vi "Counter to DAC.vi"() -> ()   [LabVIEW 2014]
uses:
  <vilib>/Platform/TimedLoop/XDataNode/timing_clust.ctl
  <vilib>/Platform/TimedLoop/XDataNode/nitl_modes.ctl
  <vilib>/Platform/TimedLoop/XDataNode/wakeup.ctl
  <vilib>/rvi/Emulation/niFpgaGetClockAttributes.vi
  <vilib>/rvi/Emulation/niFpgaSctlEmulationGetInTimedLoop.vi
  <vilib>/rvi/Emulation/niFpgaEmulationReportErrorSimple.vi
  <vilib>/rvi/Emulation/niFpgaProcessEmulError.vi
  <vilib>/rvi/Emulation/niFpgaCriticalErrorInLSC.vi
  <vilib>/rvi/interface/RandomDataEmulation/niFpgaRandomDataHandleErrors.vi
  <vilib>/rvi/eio/common/nirviEmuTemplateMethod_errors.vi
  <vilib>/Platform/TimedLoop/XDataNode/XDataNode.xnode
  <vilib>/rvi/DataTransferAndStorage/Container/XNode/niFpgaContainer.xnode
  <vilib>/rvi/interface/RandomDataEmulation/nirviRandomDataFpgaReadWriteTemplate.vi
  <vilib>/eio/EIONode/EIONode.xnode
  <vilib>/Platform/TimedLoop/XDataNode/XDNodeRunTimeDep.lvlib
panel:
  in  "ExtTrigEnable":bool
  in  "FIFOflag":bool
  out "Triggered":bool
  in  "Scale 2":i16=100
  in  "Scale 1":i16=100
  in  "Offset 2":i16
  in  "Offset 1":i16
  in  "Counter ticks":u32=40000
  out "Ctr Elapsed":u32
  out "BlocksTransfered":u32
  out "Ctr Overflow?":bool
  in  "Ctr FIFO":bool
  in  "Outputs\nDIO 12-14":bool[](array[boolean])=[FALSE, FALSE, FALSE, FALSE]
  out "Inputs\nDIO 8-10":bool[](array[boolean])=[TRUE, FALSE, FALSE]
  out "Counts":u32[](array[numeric])
  out "loop elapsed":u16
  in  "Rate":u32=400 caption="Count(Ticks)"
  out "DAC 2":i16
  out "DAC 1":i16
  in  "Dac2 sub":bool[](array[boolean])=[FALSE, FALSE, FALSE, FALSE, FALSE, FALSE, FALSE, FALSE]
  in  "Dac2 add":bool[](array[boolean])=[TRUE, TRUE, TRUE, TRUE, TRUE, TRUE, TRUE, FALSE]
  in  "Dac1 sub":bool[](array[boolean])=[FALSE, FALSE, FALSE, FALSE, FALSE, FALSE, FALSE, FALSE]
  in  "Dac1 add":bool[](array[boolean])=[TRUE, TRUE, TRUE, TRUE, TRUE, TRUE, TRUE, FALSE]
  # "Counter FIFO"
  # "Hz to Volts"
  # "TTL I/O"
  # "FPGA DMA-FIFO CANNOT be cleared by FPGA,\nonly by PC Host VI. Ctr Overflow will be on when\nFPGA-side FIFO is full!"
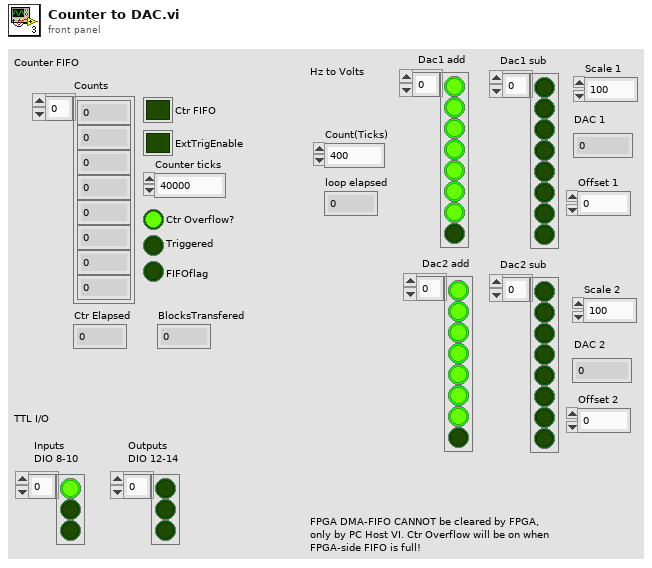
[diagram p1: front panel]
types:
  T1 = typedef "XDNodeRunTimeDep.lvlib/timing_clust.ctl" = cluster{"Expected End [f-1]":u64, "Actual End [f-1]":u64, "Finished Late? [f-1]":bool, "Expected End [i-1]":u64, "Actual End [i-1]":u64, "Finished Late? [i-1]":bool, "Expected Start [i]":u64, "Actual Start [i]":u64, "Expected Start [f]":u64, "Actual Start [f]":u64, "Source Name":string, "Structure Name":string, "Period":i64, "Deadline":i64, "Offset":i64, "Start":i64, "Priority":i32, "Timeout":i32, "Mode":T2, "Wakeup Reason":T3, "Error":errorcluster, "Source Type":string, "Secondary Source Type":string, "Global End Time":u64, "Global Start Time":u64, "Frame Duration":u64, "Iteration Duration":u64, "Assigned CPU":i32, "I/O Scan Engine Mode":u32}
  T2 = typedef "XDNodeRunTimeDep.lvlib/nitl_modes.ctl" = enum32{"No Change", "Process missed periods, maintain original phase", "Discard missed periods, maintain original phase", "Process missed periods, ignore original phase", "Discard missed periods, ignore original phase"}
  T3 = typedef "XDNodeRunTimeDep.lvlib/wakeup.ctl" = enum32{"Normal", "Aborted", "Asynchronous wakeup", "Timing source error", "Timed loop error", "Timeout"}
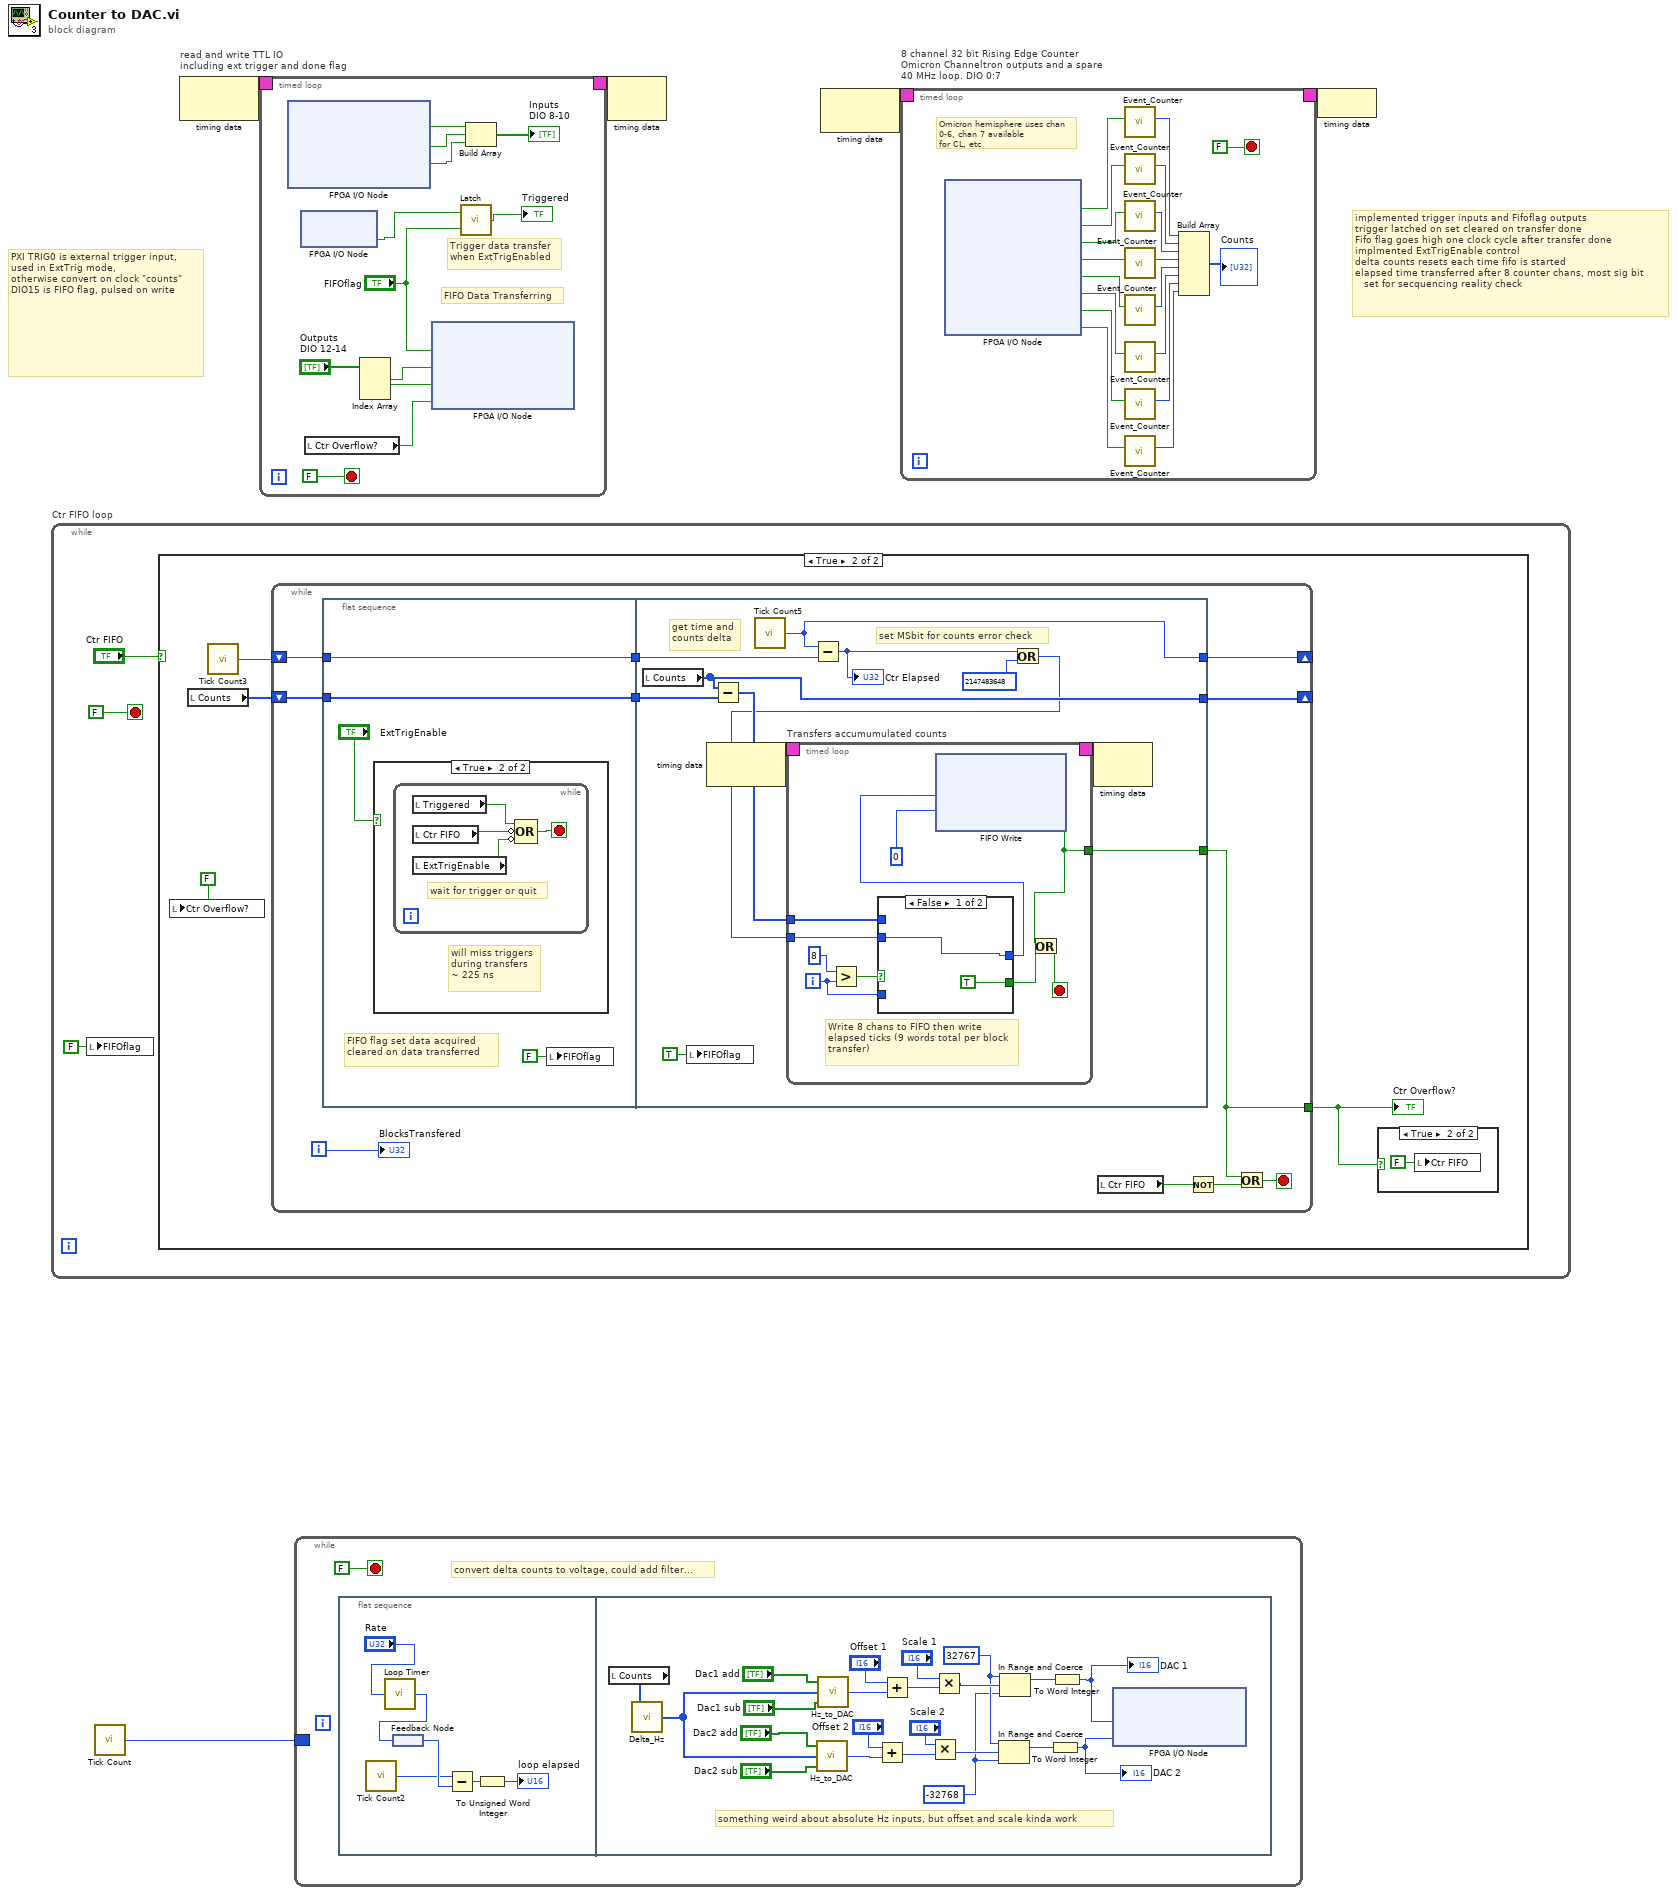
[diagram p0: block diagram]
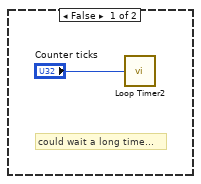
[diagram p4: hidden frame]
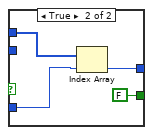
[diagram p5: hidden frame]
diagram:
  # "implemented trigger inputs and Fifoflag outputs\ntrigger latched on set cleared on transfer done\nFifo flag goes high one clock cycle after transfer done\nimplmented ExtTrigEnable control\ndelta counts resets each time fifo is started\nelapsed time transferred after 8 counter chans, most sig bit \n   set for secquencing reality check"
  # "PXI TRIG0 is external trigger input, used in ExtTrig mode, \notherwise convert on clock \"counts\"\nDIO15 is FIFO flag, pulsed on write"
  n1 = while "Ctr FIFO loop" {
    stop <- FALSE stop-if-true
    n2 = local write "FIFOflag"(FALSE ("FIFOflag")) -> ()
    n3 = case shown="True" "Ctr FIFO" {
      frame False {
      }
      frame True {
        n4 = local write "Ctr Overflow?"(FALSE ("AI Buffer Overflow?")) -> ()
        n5 = local read "Counts"() -> (w10:u32[])
        n6 = call "Tick Count3"() -> ("Tick Count(Ticks)"=w11:u32)
        n7 = while {
          shift-right: [w14] -> _
          shift-left: w11 -> [w19]
          shift-right: [w16] -> _
          shift-left: w10 -> [w17]
          tunnel: [w15] -> w9
          i -> [w21]
          stop <- w24 stop-if-true
          n8 = flat-sequence {
            tunnel: [w27] -> w20
            tunnel: w19 -> [w27]
            tunnel: [w26] -> w18
            tunnel: w17 -> [w26]
            tunnel: [w45] -> w16
            tunnel: [w35] -> w15
            tunnel: w20 -> [w41]
            tunnel: w18 -> [w40]
            tunnel: [w34] -> w14
            frame #0 {
              # "FIFO flag set data acquired cleared on data transferred"
              n9 = case shown="True" "ExtTrigEnable" {
                frame False {
                  # "could wait a long time..."
                  n10 = call "Loop Timer2"("Count(Ticks)"="Counter ticks") -> ()  [unwired: 1 out]
                }
                frame True {
                  # "will miss triggers\nduring transfers\n~ 225 ns"
                  n11 = while {
                    stop <- w33 stop-if-true
                    # "wait for trigger or quit"
                    n12 = local read "Triggered"() -> (w31:bool)
                    n13 = local read "Ctr FIFO"() -> (w30:bool)
                    n14 = local read "ExtTrigEnable"() -> (w32:bool)
                    n15 = Compound Arithmetic op=OR(w31, invert w30, invert w32) -> (w33:bool)
                  }
                }
              }
              n16 = local write "FIFOflag"(FALSE ("FIFOflag")) -> ()
            }
            frame #1 {
              # "set MSbit for counts error check"
              # "get time and\ncounts delta"
              n17 = local read "Counts"() -> (w45:u32[])
              n18 = local write "FIFOflag"(TRUE ("FIFOflag")) -> ()
              n19 = node-c288() -> (w44:T1)  [unwired: 1 in]
              n20 = Subtract(x=w45, y=w40) -> (x-y=w39:u32[])
              n21 = call "Tick Count5"() -> ("Tick Count(Ticks)"=w34:u32)
              n22 = Subtract(x=w34, y=w41) -> (x-y=w37:u32)
              "Ctr Elapsed" <- w37
              n23 = Or(x=w37, y=u32 2147483648) -> (x .or. y?=w36:u32)
              n24 = timed-loop "Transfers accumumulated counts" {
                timing: w44 -> [_]
                timing-out: [_] -> w43
                tunnel: w39 -> [w53]
                tunnel: w36 -> [w49]
                tunnel: [w47] -> w35
                i -> [w51]
                stop <- w55 stop-if-true
                # "Write 8 chans to FIFO then write elapsed ticks (9 words total per block transfer)"
                n25 = Greater?(x=8 ("y"), y=w51) -> (0:w54:bool)
                n26 = case shown="False" w54 {
                  tunnel: w53 -> [_ w61]
                  tunnel: w51 -> [_ w60]
                  tunnel: [w57 w59] -> w50
                  tunnel: w49 -> [w57 _]
                  tunnel: [TRUE ("y") FALSE ("y")] -> w46
                  frame False {
                  }
                  frame True {
                    n27 = Index Array(array=w61, index=w60) -> (element=w59:u32)
                  }
                }
                n28 = xnode ("FIFO Write")("Element"=w50, "Timeout"=0) -> ("Timed Out?"=w47:bool)  [unwired: 1 in, 1 out]
                n29 = Or(x=w47, y=w46) -> (x .or. y?=w55:bool)
              }
              n30 = node-c288(w43) -> ()  [unwired: 1 out]
            }
          }
          n31 = local read "Ctr FIFO"() -> (w23:bool)
          n32 = Not(x=w23) -> (.not. x?=w22:bool)
          n33 = Or(x=w15, y=w22) -> (x .or. y?=w24:bool)
          "BlocksTransfered" <- w21
        }
        "Ctr Overflow?" <- w9
        n34 = case shown="True" w9 {
          frame False {
          }
          frame True {
            n35 = local write "Ctr FIFO"(FALSE ("Ctr FIFO")) -> ()
          }
        }
      }
    }
  }
  n36 = call "Tick Count"() -> ("Tick Count(Ticks)"=w3:u32)
  n37 = node-c288() -> (w2:T1)  [unwired: 1 in]
  n38 = timed-loop "read and write TTL IO\nincluding ext trigger and done flag" {
    timing: w2 -> [_]
    timing-out: [_] -> w1
    stop <- FALSE stop-if-true
    # "Trigger data transfer\nwhen ExtTrigEnabled"
    # "FIFO Data Transferring"
    n39 = xnode "FPGA I/O Node"() -> ("Connector0/DIO8"=w73:bool, "Connector0/DIO9"=w75:bool, "Connector0/DIO10"=w76:bool)  [unwired: 4 in, 5 out]
    n40 = xnode "FPGA I/O Node"() -> ("TRIG0"=w66:bool)  [unwired: 1 in, 1 out]
    n41 = local read "Ctr Overflow?"() -> (w67:bool)
    n42 = Index Array(array="Outputs\nDIO 12-14") -> (element #1=w68:bool, element #2=w69:bool)  [unwired: 3 in, 1 out]
    n43 = xnode "FPGA I/O Node"("Connector0/DIO15"="FIFOflag", "Connector0/DIO12"=w68, "Connector0/DIO13"=w69, "Connector0/DIO14"=w67) -> ()  [unwired: 4 in, 4 out]
    n44 = call "Latch.vi"("reset"="FIFOflag", "set"=w66) -> ("latch"=→"Triggered":bool)
    n45 = Build Array(w73, w75, w76) -> (→"Inputs\nDIO 8-10":bool[])
  }
  n46 = while {
    border: w3 -> [_]
    stop <- FALSE stop-if-true
    # "convert delta counts to voltage, could add filter..."
    n47 = flat-sequence {
      frame #0 {
        n48 = call "Tick Count2"() -> ("Tick Count(Ticks)"=w83:u32)
        n49 = call "Loop Timer"("Count(Ticks)"="Rate") -> ("Tick Count(Ticks)"=w84:u32)
        n50 = feedback #1() -> (w86:u32)
        n51 = feedback-in #1(w84) -> ()
        n52 = Subtract(x=w83, y=w86) -> (x-y=w81:u32)
        n53 = To Unsigned Word Integer(number=w81) -> (unsigned 16bit integer=→"loop elapsed":u16)
      }
      frame #1 {
        w91 = -32768 ("lower limit")
        w92 = 32767 ("upper limit")
        # "something weird about absolute Hz inputs, but offset and scale kinda work"
        n54 = local read "Counts"() -> (w107:u32[])
        n55 = call "Delta_Hz.vi"("Counts"=w107) -> ("Delta"=w108:i32[])
        n56 = call "Hz_to_DAC.vi"("Subtract"="Dac2 sub", "Delta"=w108, "Add"="Dac2 add") -> ("Output counts"=w99:i32)
        n57 = call "Hz_to_DAC.vi"("Subtract"="Dac1 sub", "Delta"=w108, "Add"="Dac1 add") -> ("Output counts"=w102:i32)
        n58 = Add(x="Offset 2", y=w99) -> (x+y=w95:i32)
        n59 = Add(x="Offset 1", y=w102) -> (x+y=w98:i32)
        n60 = Multiply(x="Scale 2", y=w95) -> (x*y=w93:i32)
        n61 = Multiply(x="Scale 1", y=w98) -> (x*y=w94:i32)
        n62 = In Range and Coerce(upper limit=w92, x=w93, lower limit=w91) -> (coerced(x)=w88:i32)  [unwired: 1 out]
        n63 = In Range and Coerce(upper limit=w92, x=w94, lower limit=w91) -> (coerced(x)=w90:i32)  [unwired: 1 out]
        n64 = To Word Integer(number=w88) -> (16bit integer=w87:i16)
        "DAC 2" <- w87
        n65 = To Word Integer(number=w90) -> (16bit integer=w89:i16)
        "DAC 1" <- w89
        n66 = xnode "FPGA I/O Node"("Connector0/AO0"=w89, "Connector0/AO1"=w87) -> ()  [unwired: 3 in, 3 out]
      }
    }
  }
  n67 = node-c288(w1) -> ()  [unwired: 1 out]
  n68 = node-c288() -> (w5:T1)  [unwired: 1 in]
  n69 = timed-loop "8 channel 32 bit Rising Edge Counter\nOmicron Channeltron outputs and a spare\n40 MHz loop. DIO 0:7" {
    timing: w5 -> [_]
    timing-out: [_] -> w4
    stop <- FALSE stop-if-true
    # "Omicron hemisphere uses chan 0-6, chan 7 available\nfor CL, etc"
    n70 = xnode "FPGA I/O Node"() -> ("Connector0/DIO0"=w125:bool, "Connector0/DIO1"=w124:bool, "Connector0/DIO2"=w123:bool, "Connector0/DIO3"=w122:bool, "Connector0/DIO4"=w121:bool, "Connector0/DIO5"=w120:bool, "Connector0/DIO6"=w119:bool, "Connector0/DIO7"=w118:bool)  [unwired: 8 in, 8 out]
    n71 = call "Event_Counter.vi"("input"=w125) -> ("Counts"=w117:u32)  [unwired: 10 in]
    n72 = call "Event_Counter.vi"("input"=w124) -> ("Counts"=w116:u32)  [unwired: 10 in]
    n73 = call "Event_Counter.vi"("input"=w123) -> ("Counts"=w115:u32)  [unwired: 10 in]
    n74 = call "Event_Counter.vi"("input"=w122) -> ("Counts"=w114:u32)  [unwired: 10 in]
    n75 = call "Event_Counter.vi"("input"=w121) -> ("Counts"=w113:u32)  [unwired: 10 in]
    n76 = call "Event_Counter.vi"("input"=w120) -> ("Counts"=w112:u32)  [unwired: 10 in]
    n77 = call "Event_Counter.vi"("input"=w119) -> ("Counts"=w111:u32)  [unwired: 10 in]
    n78 = call "Event_Counter.vi"("input"=w118) -> ("Counts"=w110:u32)  [unwired: 10 in]
    n79 = Build Array(w117, w116, w115, w114, w113, w112, w111, w110) -> (→"Counts":u32[])
  }
  n80 = node-c288(w4) -> ()
